vi "Tester Events - Register.vi"(8 "error in":errorcluster) -> (0 "error out":errorcluster, 3 "Event Registration Refnum":refnum<event-registration>)   [LabVIEW 2024, in "Tester InterComm.lvlib"]
uses:
  Tester InterComm.lvlib
  General Actions.ctl
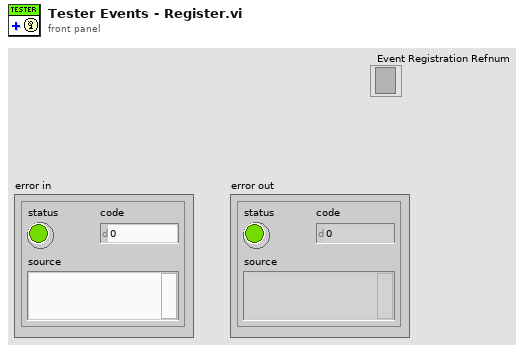
[diagram p1: front panel]
types:
  T1 = typedef "Tester InterComm.lvlib/General Actions.ctl" = enum16{"Create", "Get", "Destroy"}
  T2 = typedef "Tester InterComm.lvlib/Tester Events.ctl" = cluster{"ECU Connection Lost":refnum<user-event>, "ECU Found":refnum<user-event>}
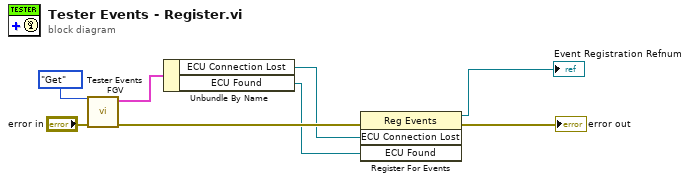
[diagram p0: block diagram]
diagram:
  n1 = call "Tester Events FGV.vi"("error in"="error in", "Action"=General_Actions."Get") -> ("error out"=w6:errorcluster, "User Events"=w4:T2)  [unwired: 8 in]
  n2 = Unbundle By Name(w4) -> ("ECU Connection Lost"=w3:refnum<user-event>, "ECU Found"=w2:refnum<user-event>)
  n3 = register-events(error in=w6, w3, w2) -> (reference out=→"Event Registration Refnum":refnum<event-registration>, error out=→"error out":errorcluster)  [unwired: 1 in]
